vi "RT_Aerodynamic_Damping_Moment (SubVI).vi"(0 "Pdin [Pa]":dbl, 1 "Data":dbl[][](array[numeric]), 2 "i":i32, 3 "V_wind [m/s]":dbl[][](array[numeric]), 4 "V(i) [m/s]":dbl[](array[numeric]), 5 "W_b(i) [rad/s]":dbl[](array[numeric]), 6 "Mach coeficients":dbl[](array[numeric]), 9 "Dref":dbl=1.72 format="%#_13g", 11 "Sref [m^2]":dbl, 13 "DCM":dbl[][](array[numeric])) -> (14 "MAd":dbl[](array[numeric]), 18 "MAd_b":dbl[](array[numeric]))   [LabVIEW 2011]
uses:
  <vilib>/Analysis/_algsub.llb/Vector Norm Type.ctl
  <vilib>/Analysis/Matrix/Numeric/Conversions/Array To Matrix - RA.vi
  <vilib>/Analysis/Matrix/Numeric/Conversions/Array To Matrix - RA2.vi
  <vilib>/Analysis/_algsub.llb/Real Vector Norm.vi
  <vilib>/Analysis/baseanly.llb/Real A x B.vi
  <vilib>/Analysis/Matrix/Numeric/Conversions/Matrix To Array - RM.vi
  <vilib>/Analysis/NI_AALPro.lvlib
  <vilib>/Analysis/NI_AALBase.lvlib
  <vilib>/Analysis/Matrix/NI_Matrix.lvlib
panel:
  out "V_norm":dbl
  out "Sref":dbl
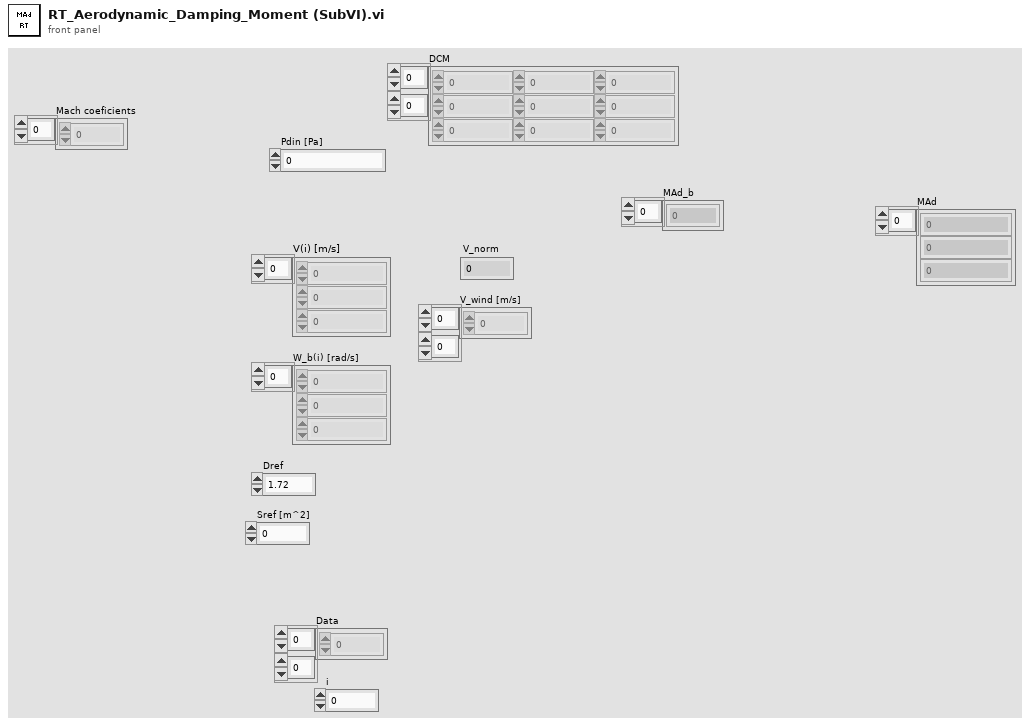
[diagram p1: front panel]
types:
  T1 = typedef "NI_AALPro.lvlib/Vector Norm Type.ctl" = u16
  T2 = typedef "NI_Matrix.lvlib/RealMatrix.ctl" = dbl[][]
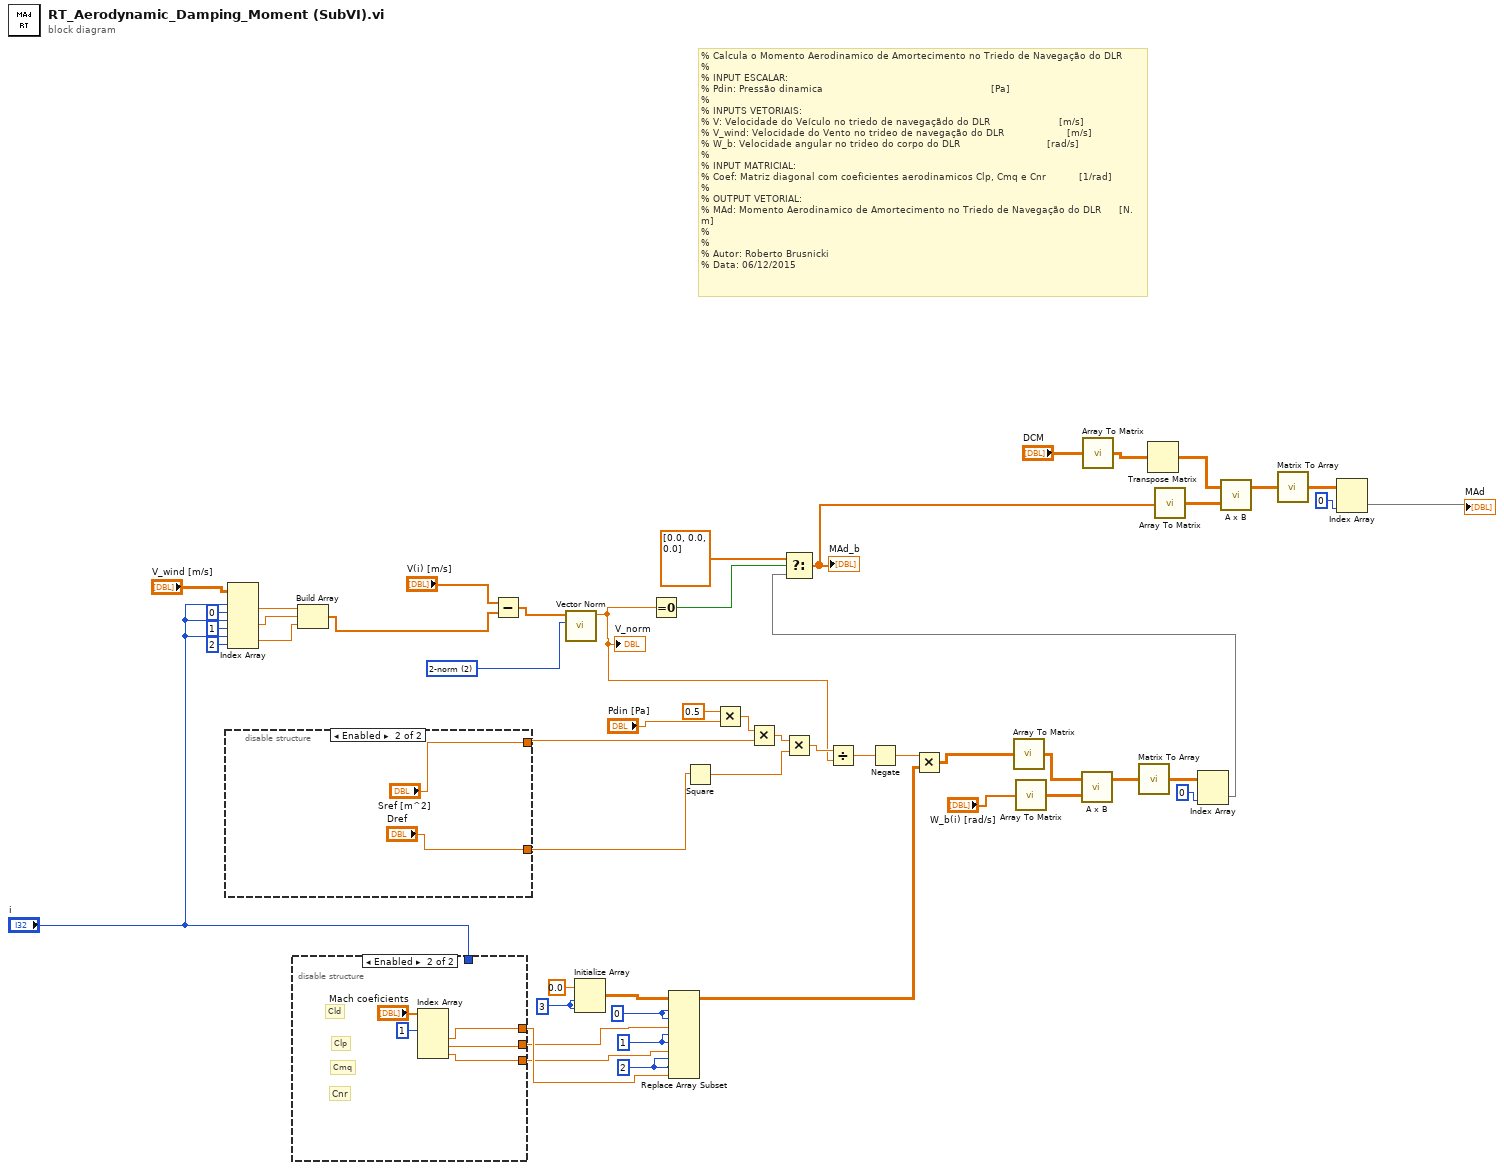
[diagram p0: block diagram]
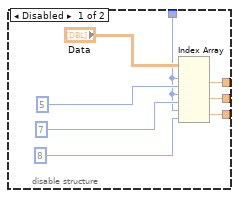
[diagram p2: hidden frame]
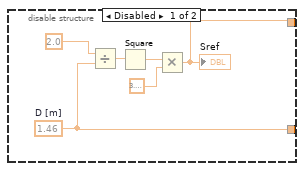
[diagram p3: hidden frame]
diagram:
  w31 = 3 ("dimension size")
  w35 = 2 ("disabled index (row)")
  w36 = 1 ("disabled index (row)")
  w34 = 0 ("disabled index (row)")
  w50 = T1 2 items=["1-norm"=1, "2-norm"=2, "Inf-norm"=3, "-Inf-norm"=4, "User Defined"=5] ("norm type")
  # "% Calcula o Momento Aerodinamico de Amortecimento no Triedo de Navegação do DLR\n%\n% INPUT ESCALAR:\n% Pdin: Pressão dinamica                                                        [Pa]\n%\n% INPUTS VETORIAIS:\n% V: Velocidade do Veículo no triedo de navegaçãdo do DLR                       [m/s]\n% V_wind: Velocidade do Vento no trideo de navegação do DLR                     [m/s]\n% W_b: Velocidade angular no trideo do corpo do DLR                             [rad/s]\n%\n% INPUT MATRICIAL:\n% Coef: Matriz diagonal com coeficientes aerodinamicos Clp, Cmq e Cnr           [1/rad]\n%\n% OUTPUT VETORIAL:\n% MAd: Momento Aerodinamico de Amortecimento no Triedo de Navegação do DLR      [N.m]\n% \n%\n% Autor: Roberto Brusnicki\n% Data: 06/12/2015"
  n1 = disable-structure shown="Enabled" {
    disable-tunnel: [w54 "Dref"] -> w44
    disable-tunnel: [w53 "Sref [m^2]"] -> w42
    frame Disabled {
      w54 = 1.46  # D [m]
      n2 = Divide(x=2.0 ("y"), y=w54) -> (x/y=w56:dbl)
      n3 = Square(x=w56) -> (x^2=w57:dbl)
      n4 = Multiply(x=w57, y=3.141592653589793) -> (x*y=w53:dbl)
      "Sref" <- w53
    }
    frame Enabled {
    }
  }
  n5 = Index Array(array="V_wind [m/s]", index (row) #1="i", index (col) #1=0 ("disabled index (col)"), index (row) #2="i", index (col) #2=1 ("disabled index (col)"), index (row) #3="i", index (col) #3=2 ("disabled index (col)")) -> (element #1=w8:dbl, element #2=w7:dbl, element #3=w6:dbl)
  n6 = disable-structure shown="Enabled" {
    disable-tunnel: [w64 w71] -> w3
    disable-tunnel: [w63 w70] -> w1
    disable-tunnel: [w62 w69] -> w2
    disable-tunnel: "i" -> [w61 _]
    frame Disabled {
      n7 = Index Array(array="Data", index (row) #1=w61, index (col) #1=5 ("disabled index (col)"), index (row) #2=w61, index (col) #2=7 ("disabled index (col)"), index (row) #3=w61, index (col) #3=8 ("disabled index (col)")) -> (element #1=w64:dbl, element #2=w63:dbl, element #3=w62:dbl)
    }
    frame Enabled {
      # "Cnr"
      # "Cmq"
      # "Clp"
      # "Cld"
      n8 = Index Array(array="Mach coeficients", index #1=1 ("index")) -> (element #2=w71:dbl, element #3=w70:dbl, element #4=w69:dbl)  [unwired: 3 in, 1 out]
    }
  }
  n9 = Build Array(w8, w7, w6) -> (w5:dbl[])
  n10 = Subtract(x="V(i) [m/s]", y=w5) -> (x-y=w51:dbl[])
  n11 = call-poly <vilib>:"Vector Norm.vi"("norm type"=w50, "Input Vector"=w51) -> ("norm"=w39:dbl)  [unwired: 8 in, 1 out]
  "V_norm" <- w39
  n12 = Initialize Array(0.0 ("element"), w31, w31) -> (w33:dbl[][])
  n13 = Equal To 0?(x=w39) -> (x = 0?=w49:bool)
  n14 = Replace Array Subset(array=w33, new element #1=w1, index (row) #1=w34, index (col) #1=w34, new element #2=w2, index (row) #2=w36, index (col) #2=w36, new element #3=w3, index (row) #3=w35, index (col) #3=w35) -> (w30:dbl[][])
  n15 = Square(x=w44) -> (x^2=w43:dbl)
  n16 = Multiply(x=0.5, y="Pdin [Pa]") -> (x*y=w47:dbl)
  n17 = Multiply(x=w47, y=w42) -> (x*y=w46:dbl)
  n18 = Multiply(x=w46, y=w43) -> (x*y=w45:dbl)
  n19 = Divide(x=w45, y=w39) -> (x/y=w38:dbl)
  n20 = Negate(x=w38) -> (-x=w37:dbl)
  n21 = Multiply(x=w37, y=w30) -> (x*y=w25:dbl[][])
  n22 = call-poly <vilib>:"Array To Matrix.vi"("Real 2D Array"=w25) -> ("Real Matrix"=w24:T2)
  n23 = call-poly <vilib>:"Array To Matrix.vi"("Real 1D Array"="W_b(i) [rad/s]") -> ("Real Matrix (Column Vector)"=w29:T2)
  n24 = call-poly <vilib>:"A x B.vi"("B"=w29, "A"=w24) -> ("A x B"=w27:T2)  [unwired: 1 out]
  n25 = call-poly <vilib>:"Array To Matrix.vi"("Real 2D Array"="DCM") -> ("Real Matrix"=w16:T2)
  n26 = call-poly <vilib>:"Matrix To Array.vi"("Real Matrix"=w27) -> ("Real 2D Array"=w28:dbl[][])
  n27 = Transpose Matrix(1:w16) -> (0:w15:T2)
  n28 = Index Array(array=w28, index (col)=0 ("index (row)")) -> (element=w22:dbl[])  [unwired: 1 in]
  n29 = Select(t=dbl[] [0.0, 0.0, 0.0] ("V_wind [m/s] 2"), s=w49, f=w22) -> (s? t:f=w14:dbl[])
  "MAd_b" <- w14
  n30 = call-poly <vilib>:"Array To Matrix.vi"("Real 1D Array"=w14) -> ("Real Matrix (Column Vector)"=w21:T2)
  n31 = call-poly <vilib>:"A x B.vi"("B"=w21, "A"=w15) -> ("A x B"=w19:T2)  [unwired: 1 out]
  n32 = call-poly <vilib>:"Matrix To Array.vi"("Real Matrix"=w19) -> ("Real 2D Array"=w20:dbl[][])
  n33 = Index Array(array=w20, index (col)=0 ("index (row)")) -> (element=→"MAd":dbl[])  [unwired: 1 in]
